vi "Set State.vi"(8 "error in (no error)":errorcluster, 10 "Output":T1, 11 "RP100 in":refnum<class "RP100.lvclass">) -> (0 "error out":errorcluster, 3 "RP100 out":refnum<class "RP100.lvclass">)   [LabVIEW 2019, in "RP100.lvclass"]
doc: "Set the output <b>Level</b> with <b>Slew</b> rate on the selected <b>Output Channel</b>"
uses:
  RP100.lvclass
  C:/Program Files (x86)/National Instruments/LabVIEW 2019/user.lib/LevyLab/Instrument Framework/SMOs/Instrument/Instrument.lvclass
  Typedefs/Output State--Enum.ctl
  Typedefs/Commands--Enum.ctl
  Typedefs/setOutput--Cluster.ctl
  <userlib>/LevyLab/Instrument Framework/SMOs/Instrument/Instrument.lvclass/Instrument.ctl
  561c9bc1-5633-4095-b2f1-945bf898e835.vi
  Set Output.vi/561c9bc1-5633-4095-b2f1-945bf898e835.vi/fb75245c-0d96-46ba-a325-ca721577eb16.vi
  Set Output.vi/561c9bc1-5633-4095-b2f1-945bf898e835.vi/fb75245c-0d96-46ba-a325-ca721577eb16.vi/f21d0bf1-848c-4cc8-ba1f-f946bbc9d011.vi
  <userlib>/LevyLab/Instrument Framework/SMOs/Instrument/API/Send and Receive.vi
  Set Output.vi/561c9bc1-5633-4095-b2f1-945bf898e835.vi/fb75245c-0d96-46ba-a325-ca721577eb16.vi/f21d0bf1-848c-4cc8-ba1f-f946bbc9d011.vi/a2560186-1067-4110-8c1b-103b06b7b896.vi
  Set Output.vi/561c9bc1-5633-4095-b2f1-945bf898e835.vi/fb75245c-0d96-46ba-a325-ca721577eb16.vi/f21d0bf1-848c-4cc8-ba1f-f946bbc9d011.vi/9cfc5259-0444-4612-9b27-6efe563139f8.vi
  <userlib>/LevyLab/Instrument Framework/SMOs/Instrument/API/Enum to String.vi
  <userlib>/LevyLab/Instrument Framework/SMOs/RemoteControl/API/Send and Receive.vi
  <vilib>/Utility/Data Type/Get Type Information.vi
  <vilib>/JDP Science/JSONtext/JSON text to Variant.vi
  <vilib>/JDP Science/JSONtext/LVClass Serializer/JSONtext LVClass Serializer.lvclass
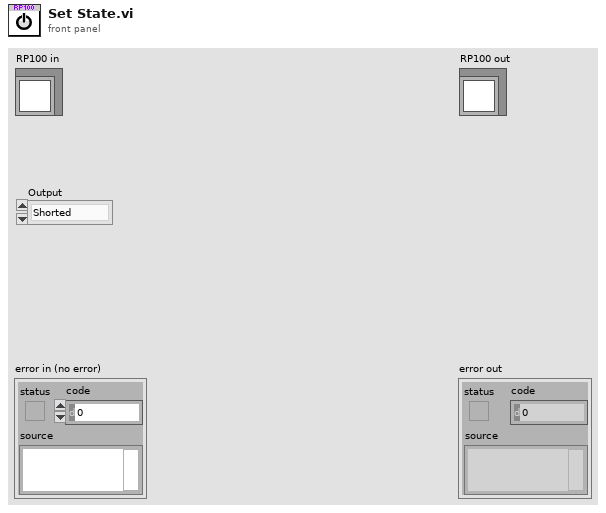
[diagram p1: front panel]
types:
  T1 = typedef "RP100.lvclass/Output State--Enum.ctl" = enum16{"Shorted", "Enabled"}
  T2 = typedef "RP100.lvclass/setOutput--Cluster.ctl" = cluster{"State":T1}
  T3 = typedef "RP100.lvclass/Commands--Enum.ctl" = enum16{"setState", "setStrain", "getStrain", "setLevel", "getLevel"}
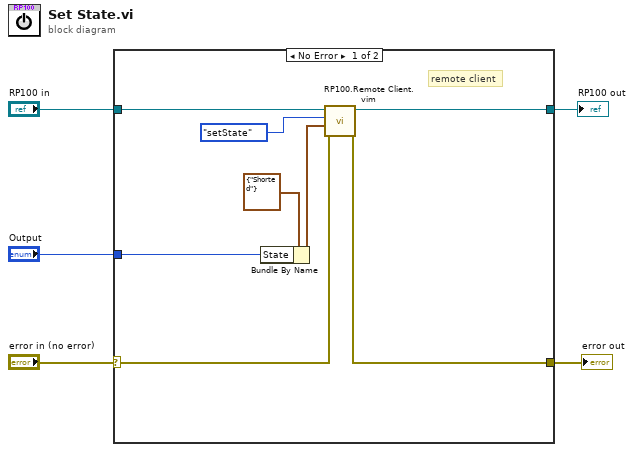
[diagram p0: block diagram]
diagram:
  n1 = case shown="No Error" "error in (no error)" {
    selector: "error in (no error)" -> [w11 w15]
    tunnel: [w10 w15] -> w4
    tunnel: "Output" -> [w7 _]
    tunnel: "RP100 in" -> [w13 w14]
    tunnel: [w12 w14] -> w1
    frame No Error {
      # "remote client"
      n2 = Bundle By Name(cluster=T2 {"State"=enum."Shorted"} ("setOutput"), "State"=w7) -> (w8:T2)
      n3 = call "RP100.Remote Client.vim"("error in (no error)"=w11, "params"=w8, "Commands"=Commands--Enum."setState", "RP100 in"=w13) -> ("error out"=w10:errorcluster, "RP100 out"=w12:refnum<class "RP100.lvclass">)  [unwired: 5 in, 1 out]
    }
    frame Error {
    }
  }
  "error out" <- w4
  "RP100 out" <- w1
